vi "External Actuator Channel Names DAO.vi"(7 "refnum":T2, 8 "error in (no error)":errorcluster, 9 "External Actuator Id":T1, 10 "DAQ Channel In":T3, 11 "Persistent DAO Actions":T4) -> (0 "error out":errorcluster, 2 "DAQ Channel Out":T3, 4 "refnum out":T2)   [LabVIEW 2009]
uses:
  Metadata/Persistant DAO Actions.ctl
  External Actuator Channels.ctl
  <vilib>/Utility/config.llb/Config Data RefNum.ctl
  External Actuator Id.ctl
  <vilib>/Utility/config.llb/NI_LVConfig.lvlib
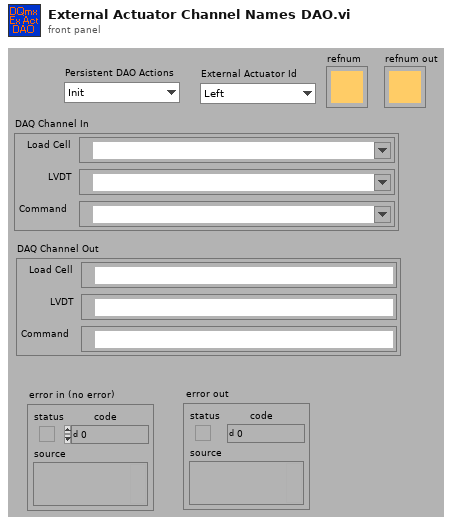
[diagram p1: front panel]
types:
  T1 = typedef "External Actuator Id.ctl" = enum16{"Left", "Right"}
  T2 = typedef "NI_LVConfig.lvlib/Config Data RefNum.ctl" = refnum<k1>
  T3 = typedef "External Actuator Channels.ctl" = cluster{"Load Cell":refnum<k21>, "LVDT":refnum<k21>, "Command":refnum<k21>}
  T4 = typedef "Persistant DAO Actions.ctl" = enum16{"Init", "Get", "Set", "Load", "Save"}
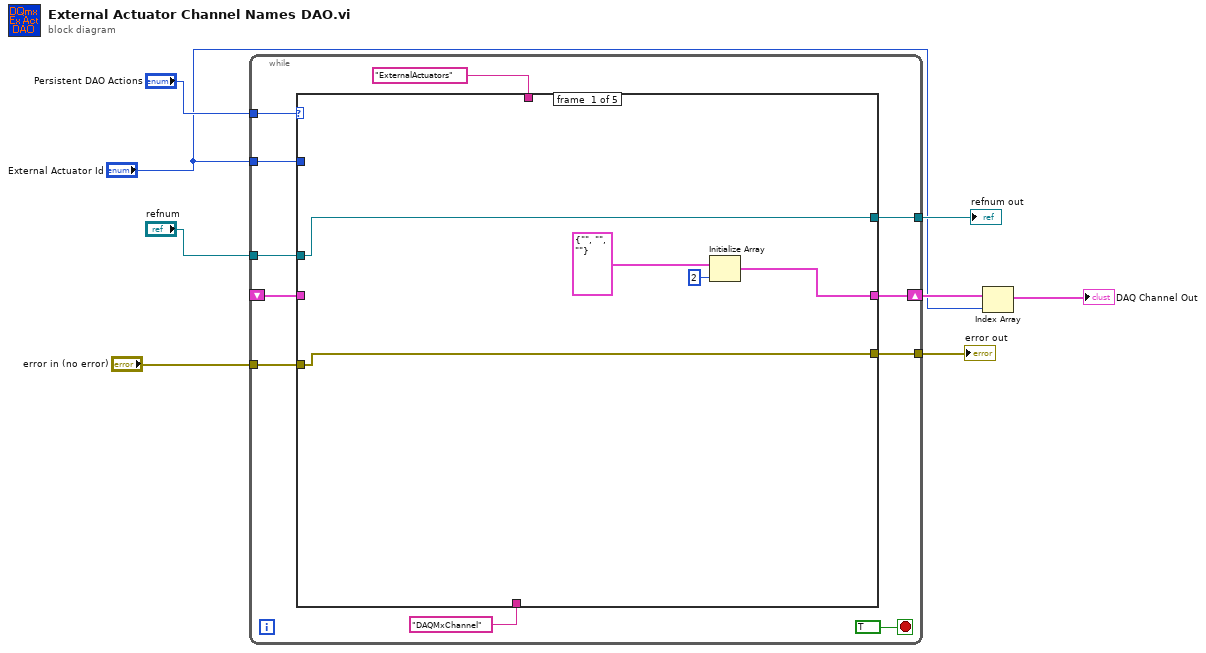
[diagram p0: block diagram]
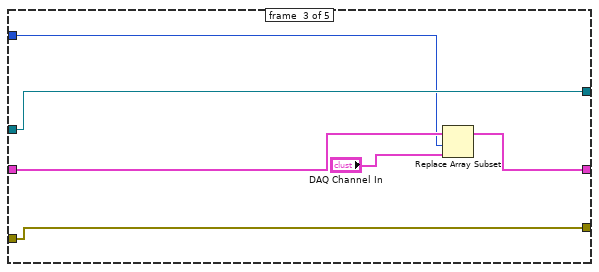
[diagram p3: hidden frame]
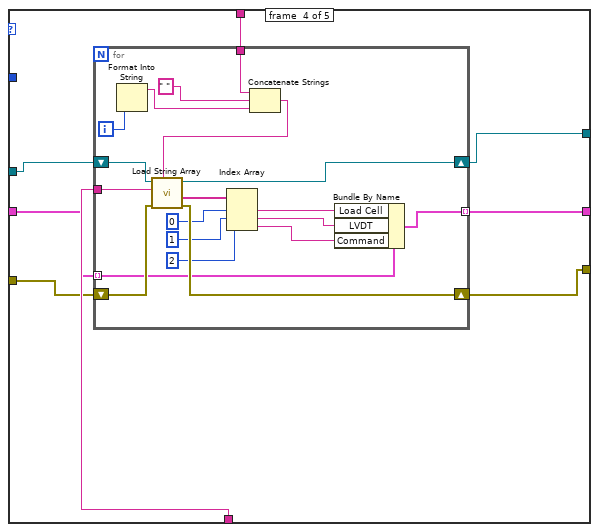
[diagram p4: hidden frame]
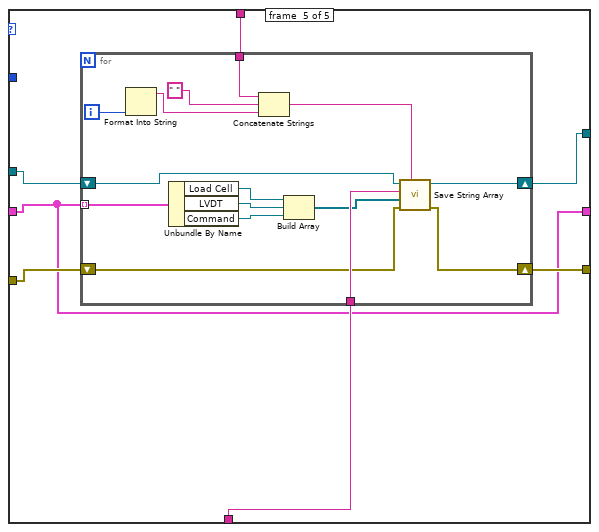
[diagram p5: hidden frame]
diagram:
  n1 = while {
    tunnel: "Persistent DAO Actions" -> [w18]
    shift-right: [w17] -> w7
    shift-left: _ -> [w16]
    tunnel: "refnum" -> [w15]
    tunnel: "error in (no error)" -> [w12]
    tunnel: [w11] -> w4
    tunnel: [w10] -> w3
    tunnel: "External Actuator Id" -> [w9]
    stop <- TRUE stop-if-true
    n2 = case shown="\"Load\"" w18 {
      tunnel: [w21 w27 w31 w34 w61] -> w17
      tunnel: w16 -> [_ w27 w29 w35 w61]
      tunnel: w15 -> [w23 w26 w33 w39 w67]
      tunnel: "DAQMxChannel" -> [_ _ _ w41 w66]
      tunnel: "ExternalActuators" -> [_ _ _ w40 w65]
      tunnel: w12 -> [w22 w25 w32 w37 w64]
      tunnel: [w23 w26 w33 w38 w63] -> w11
      tunnel: [w22 w25 w32 w36 w62] -> w10
      tunnel: w9 -> [_ _ w28 _ _]
      frame #0 {
        n3 = Initialize Array(T3 {"Load Cell"="", "LVDT"="", "Command"=""} ("DAQ Channel In"), 2 ("dimension size")) -> (w21:T3[])
      }
      frame #1 {
      }
      frame #2 {
        n4 = Replace Array Subset(array=w29, new element="DAQ Channel In", index=w28) -> (w31:T3[])
      }
      frame #3 {
        n5 = for {
          tunnel: w41 -> [w60]
          tunnel: w40 -> [w43]
          tunnel: w35 -> [w51] mode=indexing
          tunnel: [w47] -> w34 mode=indexing
          shift-right: [w58] -> w38
          shift-left: w39 -> [w59]
          shift-right: [w56] -> w36
          shift-left: w37 -> [w57]
          i -> [w42]
          n6 = Format Into String(w42) -> (resulting string=w46:string)  [unwired: 3 in, 1 out]
          n7 = Concatenate Strings(w43, " " ("string"), w46) -> (w44:string)
          n8 = call "Load String Array.vi"("section"=w44, "error in (no error)"=w57, "key"=w60, "refnum"=w59) -> ("error out"=w56:errorcluster, "String Array Out"=w55:string[], "refnum out"=w58:T2)  [unwired: 5 out]
          n9 = Index Array(array=w55, index #1=0 ("index"), index #2=1 ("index"), index #3=2 ("index")) -> (element #1=w50:string, element #2=w49:string, element #3=w48:string)
          n10 = Bundle By Name(cluster=w51, "Load Cell"=w50, "LVDT"=w49, "Command"=w48) -> (w47:T3)
        }
      }
      frame #4 {
        n11 = for {
          tunnel: w66 -> [w81]
          tunnel: w65 -> [w69]
          tunnel: w61 -> [w77] mode=indexing
          shift-right: [w78] -> w62
          shift-left: w64 -> [w80]
          shift-right: [w79] -> w63
          shift-left: w67 -> [w82]
          i -> [w70]
          n12 = Format Into String(w70) -> (resulting string=w72:string)  [unwired: 3 in, 1 out]
          n13 = Unbundle By Name(w77) -> ("Load Cell"=w76:refnum<k21>, "LVDT"=w74:refnum<k21>, "Command"=w73:refnum<k21>)
          n14 = Concatenate Strings(w69, " " ("string"), w72) -> (w68:string)
          n15 = Build Array(w76, w74, w73) -> (w75:refnum<k21>[])
          n16 = call "Save String Array.vi"("section"=w68, "error in (no error)"=w80, "String Array In"=w75, "key"=w81, "refnum"=w82) -> ("error out"=w78:errorcluster, "refnum out"=w79:T2)  [unwired: 5 out]
        }
      }
    }
  }
  "refnum out" <- w4
  "error out" <- w3
  n17 = Index Array(array=w7, index="External Actuator Id") -> (element=→"DAQ Channel Out":T3)
